vi "Корректировка.vi"() -> ()   [LabVIEW 2011]
uses:
  granula_llb.lvlib
panel:
  in  "Тек. В":dbl
  in  "Тек. А":dbl
  in  "Закрыть окно":bool
  in  "Сохранить":bool
  in  "ВЫЧЕСТЬ":bool
  in  "B":dbl
  in  "A":dbl
  # "T=T+A+T*B"
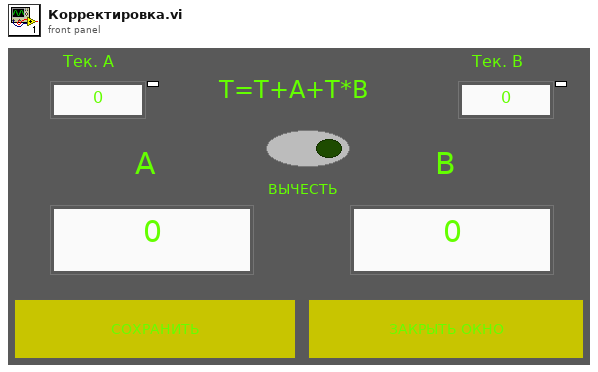
[diagram p1: front panel]
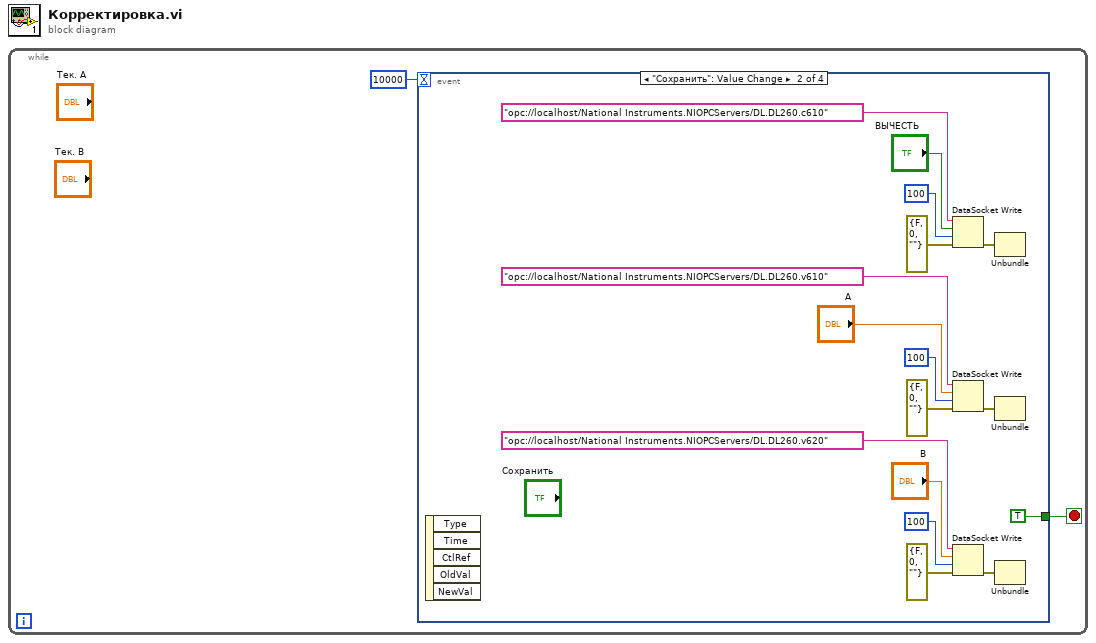
[diagram p0: block diagram]
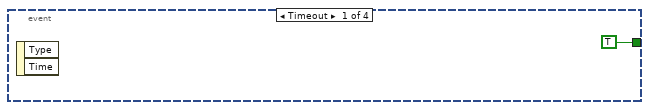
[diagram p2: hidden frame]
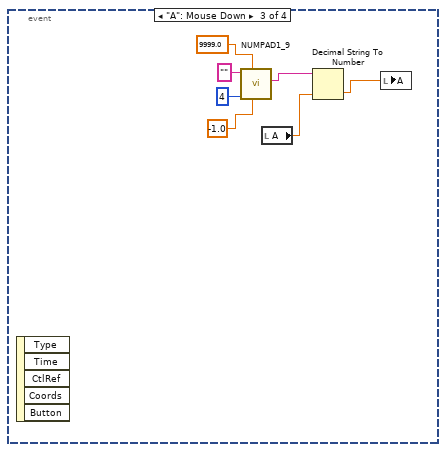
[diagram p3: hidden frame]
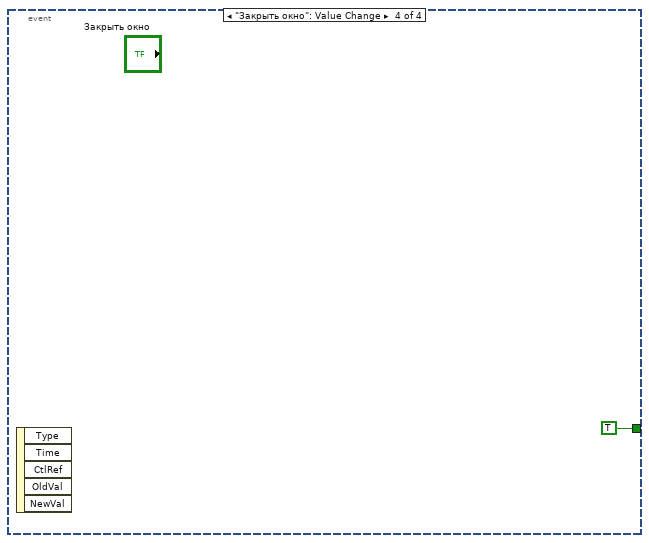
[diagram p4: hidden frame]
diagram:
  n1 = while {
    stop <- w1 stop-if-true
    n2 = event shown="[1] \"Сохранить\": Value Change" {
      selector: _ -> [_ _ _ _]
      dyn-events: _ -> [_ _ _ _]
      timeout: 10000 -> [_ _ _ _]
      tunnel: [TRUE TRUE _ TRUE] -> w1
      event Timeout {
        n3 = event-data() -> ()  [unwired: 1 in, 2 out]
      }
      event "Сохранить": Value Change {
        n4 = event-data() -> ()  [unwired: 1 in, 5 out]
        n5 = DataSocket Write(8:errorcluster {"status"=FALSE, "code"=0, "source"=""} ("error in (no error)"), 9:100 ("ms timeout (0)"), 10:"ВЫЧЕСТЬ", 11:"opc://localhost/National Instruments.NIOPCServers/DL.DL260.c610" ("connection in")) -> (0:w4:errorcluster)  [unwired: 2 out]
        n6 = DataSocket Write(8:errorcluster {"status"=FALSE, "code"=0, "source"=""} ("error in (no error)"), 9:100 ("ms timeout (0)"), 10:"A", 11:"opc://localhost/National Instruments.NIOPCServers/DL.DL260.v610" ("connection in")) -> (0:w9:errorcluster)  [unwired: 2 out]
        n7 = DataSocket Write(8:errorcluster {"status"=FALSE, "code"=0, "source"=""} ("error in (no error)"), 9:100 ("ms timeout (0)"), 10:"B", 11:"opc://localhost/National Instruments.NIOPCServers/DL.DL260.v620" ("connection in")) -> (0:w14:errorcluster)  [unwired: 2 out]
        n8 = Unbundle(w4) -> ()  [unwired: 3 out]
        n9 = Unbundle(w9) -> ()  [unwired: 3 out]
        n10 = Unbundle(w14) -> ()  [unwired: 3 out]
      }
      event "A": Mouse Down {
        n11 = event-data() -> ()  [unwired: 1 in, 5 out]
        n12 = call "NUMPAD1_9.vi"("МИНИМАЛЬНОЕ ЗНАЧЕНИЕ"=-1.0, "МАКСИМАЛЬНОЕ ЗНАЧЕНИЕ"=9999.0, "ДЛИННА СЛОВА"=i8 4, "ТЕКУЩЕЕ ЗНАЧЕНИЕ"="") -> ("НОВОЕ ЗНАЧЕНИЕ"=w22:string)  [unwired: 7 in]
        n13 = local read "A"() -> (w21:dbl)
        n14 = Decimal String To Number(string=w22, default (0L)=w21) -> (number=w20:dbl)  [unwired: 1 in, 1 out]
        n15 = local write "A"(w20) -> ()
      }
      event "Закрыть окно": Value Change {
        n16 = event-data() -> ()  [unwired: 1 in, 5 out]
      }
    }
  }
